vi "XNodeStateMessage.vi"() -> ()   [LabVIEW 2010]
uses:
  XStateMessage.ctl
  CThread/XNodes/referencenode/State.ctl
  CThread/XNodes/referencenode/CThread VI Reference.xnode
panel:
  in  "State":T1={"VI Name"="", "VI Path"=path "", "Clone"=0, "Encoded Name"=0, "XStateMessage"={"Hook"="sdfsdfsdf", "Length"=0, "Reply?"=FALSE, "Data"=""}}
  out "found":bool
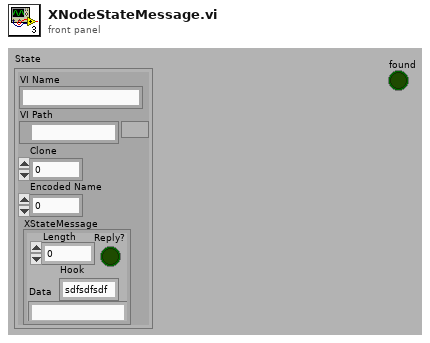
[diagram p1: front panel]
types:
  T1 = typedef "CThread.lvlib/CThread VI Reference.xnode/State.ctl" = cluster{"VI Name":string, "VI Path":path, "Clone":i16, "Encoded Name":u32, "XStateMessage":T2}
  T2 = typedef "XStateMessage.ctl" = cluster{"Hook":string, "Length":u16, "Reply?":bool, "Data":string}
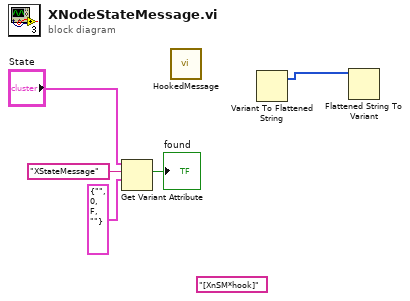
[diagram p0: block diagram]
diagram:
  (unwired) "[XnSM*hook]"
  n1 = Get Variant Attribute(Variant="State", name="XStateMessage", default value (empty Variant)=T2 {"Hook"="", "Length"=0, "Reply?"=FALSE, "Data"=""} ("XStateMessage")) -> (found=→"found":bool)  [unwired: 1 in, 3 out]
  n2 = call "HookedMessage.vi"() -> ()  [unwired: 7 in, 2 out]
  n3 = Variant To Flattened String() -> (1:w1:i16[])  [unwired: 1 in, 1 out]
  n4 = Flattened String To Variant(7:w1) -> ()  [unwired: 2 in, 2 out]
